vi "GetGlobalReference.vi"(8 "error in (no error)":errorcluster) -> (0 "error out":errorcluster, 3 "reference":T1)   [LabVIEW 2017, in "DVRBuffer.lvlib"]
uses:
  <vilib>/addons/InsightCM/Devices/Shared/Common/DVRBuffer/DVRBuffer.lvlib
  <vilib>/addons/PointValueMap/controls/PointMap.ctl
  <vilib>/addons/PointValueMap/PointValueMap.lvlib
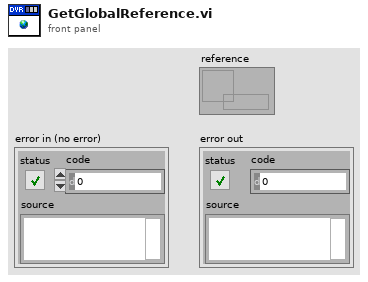
[diagram p1: front panel]
types:
  T1 = typedef "PointValueMap.lvlib/PointMap.ctl" = refnum<data-value>
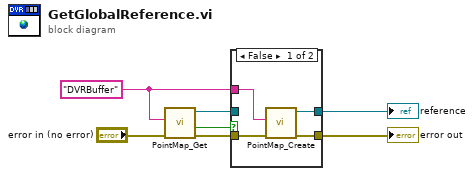
[diagram p0: block diagram]
diagram:
  w5 = "DVRBuffer" ("Name")
  n1 = call <vilib>:"PointMap_Get.vi"("error in (no error)"="error in (no error)", "Name"=w5) -> ("error out"=w3:errorcluster, "Found?"=w2:bool, "Map Out"=w4:T1)  [unwired: 7 in]
  n2 = case shown="False" w2 {
    tunnel: w3 -> [w11 w12]
    tunnel: w4 -> [_ w13]
    tunnel: w5 -> [w10 _]
    tunnel: [w9 w12] -> w6
    tunnel: [w8 w13] -> w7
    frame False {
      n3 = call <vilib>:"PointMap_Create.vi"("error in (no error)"=w11, "Name"=w10) -> ("error out"=w9:errorcluster, "Map Out"=w8:T1)  [unwired: 8 in]
    }
    frame True {
    }
  }
  "reference" <- w7
  "error out" <- w6
